vi "test_python_installation.vi"() -> ()   [LabVIEW 2011]
panel:
  out "error out 2":errorcluster
  out "error out":errorcluster
  in  "error in (no error)":errorcluster
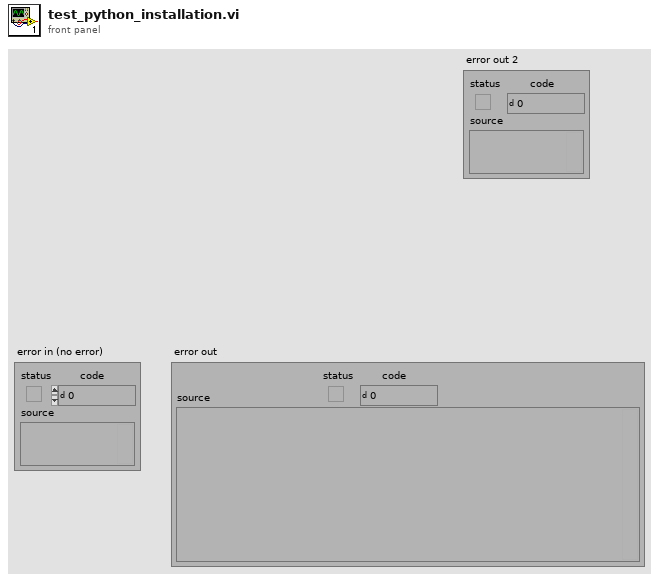
[diagram p1: front panel]
types:
  T1 = typedef "PYTHON Session Refnum__ogtk.ctl" = refnum<k1>
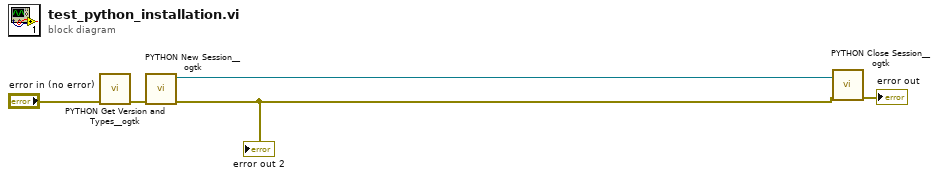
[diagram p0: block diagram]
diagram:
  n1 = call <userlib>:"PYTHON Get Version and Types__ogtk.vi"("error in (no error)"="error in (no error)") -> ("error out"=w5:errorcluster)  [unwired: 4 in, 2 out]
  n2 = call <userlib>:"PYTHON New Session__ogtk.vi"("error in (no error)"=w5) -> ("error out"=w1:errorcluster, "Python Session"=w2:T1)  [unwired: 5 in]
  "error out 2" <- w1
  n3 = call <userlib>:"PYTHON Close Session__ogtk.vi"("error in (no error)"=w1, "Python Session in"=w2) -> ("error out"=→"error out":errorcluster)  [unwired: 5 in]
